vi "get_observers.vi"(8 "error in (no error)":errorcluster, 11 "GenericToplevelComponent in":refnum<class "GenericToplevelComponent.lvclass">) -> (0 "error out":errorcluster, 2 "observers":refnum<class "GenericToplevelComponent.lvclass">[](array[class]), 3 "GenericToplevelComponent out":refnum<class "GenericToplevelComponent.lvclass">)   [LabVIEW 2010, in "GenericToplevelComponent.lvclass"]
uses:
  GenericToplevelComponent.lvclass
  GenericToplevelComponent.lvclass/GenericToplevelComponent.ctl
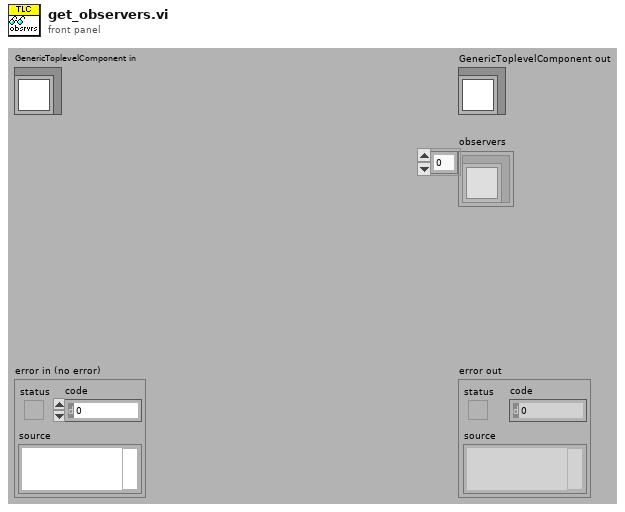
[diagram p1: front panel]
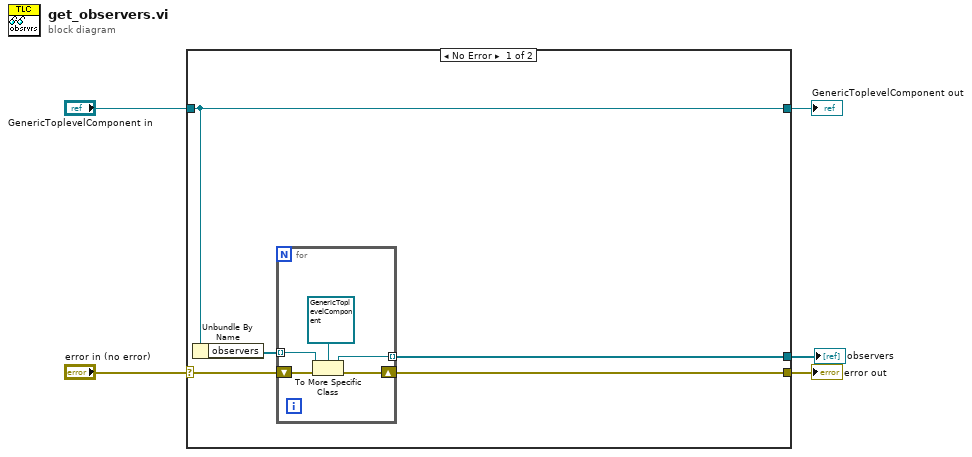
[diagram p0: block diagram]
diagram:
  n1 = case shown="No Error" "error in (no error)" {
    selector: "error in (no error)" -> [w10 w17]
    tunnel: [w9 w17] -> w4
    tunnel: [w8 w16] -> w2
    tunnel: "GenericToplevelComponent in" -> [w8 w16]
    tunnel: [w6 _] -> w1
    frame No Error {
      n2 = Unbundle By Name(w8) -> ("observers"=w7:refnum<class "GenericComponent.lvclass">[])
      n3 = for {
        shift-right: [w13] -> w9
        shift-left: w10 -> [w14]
        tunnel: w7 -> [w12] mode=indexing
        tunnel: [w11] -> w6 mode=indexing
        n4 = To More Specific Class(target class=refnum<class "GenericToplevelComponent.lvclass"> refnum ("GenericToplevelComponent.lvclass"), reference=w12, error in=w14) -> (specific class reference=w11:refnum<class "GenericToplevelComponent.lvclass">, error out=w13:errorcluster)
      }
    }
    frame Error {
    }
  }
  "error out" <- w4
  "GenericToplevelComponent out" <- w2
  "observers" <- w1
